vi "Periodic Tasks.vi"(8 "error in":errorcluster) -> ()   [LabVIEW 2017]
doc: "This VI runs in parallel to other robot code. It can contain as many user-defined periodic loops as you need. These can carry out PID or other sorts of timed response."
uses:
  2018_Trobots_5013_Dashboard/Routines and Block Data.ctl
  Support Code/Blocks.ctl
  <vilib>/Rock Robotics/Network Tables/NT Read Boolean.vi
  Robot Global Data.vi
  <vilib>/Rock Robotics/Network Tables/NT Write Boolean.vi
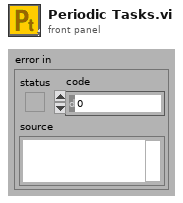
[diagram p1: front panel]
types:
  T1 = typedef "Routines and Block Data.ctl" = cluster{"Routines":T2[][], "Block Data Array":variant[]}
  T2 = typedef "Blocks.ctl" = enum16{"", "Wait 1s", "Far to L1", "L1 to End Switch 1", "End Switch 1 to C1", "End Cube to C1", "C1 to Diag Scale 1", "C1 to C3", "C3 to C4", "Diag Scale to C1", "C3 to End Switch 2", "C4 to Diag Scale 2", "C3 to Cube&Switch", "Middle to Front S2", "Middle to Front S1", "Front S1 to Line 1", "Front S2 to Line 2", "End Switch 1 to End Cube", "Line 1 to C1"}
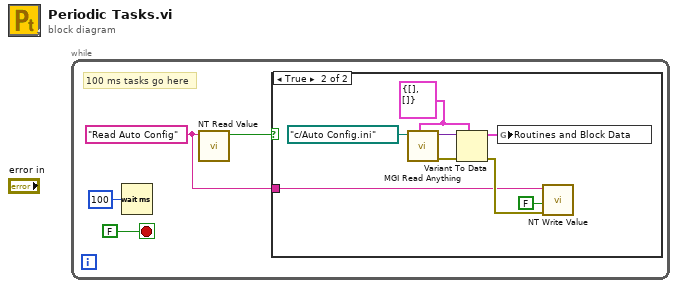
[diagram p0: block diagram]
diagram:
  n1 = while {
    stop <- FALSE stop-if-true
    w1 = "Read Auto Config" ("Name")
    # "100 ms tasks go here"
    n2 = Wait (ms)(milliseconds to wait=u32 100) -> ()  [unwired: 1 out]
    n3 = call-poly <vilib>:"NT Read Value.vi"("Name"=w1) -> ("Boolean"=w2:bool)  [unwired: 9 in, 1 out]
    n4 = case shown="True" w2 {
      tunnel: w1 -> [_ w7]
      frame False {
      }
      frame True {
        w10 = T1 {"Routines"=[], "Block Data Array"=[]} ("Routines and Block Data")
        n5 = call <userlib>:"MGI Read Anything.vi"("Type of Anything"=w10, "Path (dialog)"=path "c:/Auto Config.ini") -> ("Error Out"=w12:errorcluster, "Anything"=w11:variant)  [unwired: 6 in, 2 out]
        n6 = Variant To Data(error in=w12, type=w10, Variant=w11) -> (data=w9:T1, error out=w8:errorcluster)
        n7 = global write "Robot Global Data.vi" "Routines and Block Data"(w9) -> ()
        n8 = call-poly <vilib>:"NT Write Value.vi"("error in"=w8, "Boolean"=FALSE, "Name"=w7) -> ()  [unwired: 8 in, 1 out]
      }
    }
  }
